vi "FTP Directory check Create if needed.vi"(0 "Host":string, 1 "Create dir":bool, 5 "UserName":string, 7 "Password":string, 9 "PathToCreate":string, 11 "error in (no error)":errorcluster, 12 "timeout ms (60000)":i32=60000) -> (10 "Path":string, 15 "error out":errorcluster)   [LabVIEW 2010]
doc: "This VI checks to see if an FTP file path exists, and if it doesn't then creates it"
uses:
  <vilib>/addons/internet/NI_InternetTK_FTP_VIs.lvlib
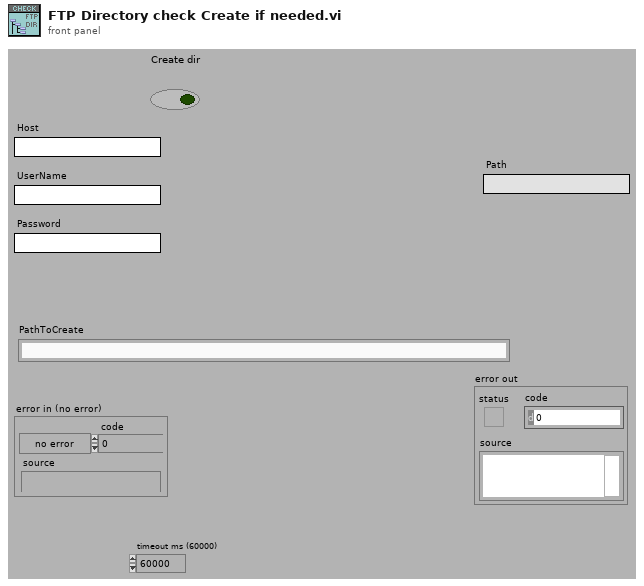
[diagram p1: front panel]
types:
  T1 = typedef "FTP Session.ctl" = refnum<k1>
  T2 = typedef "FTP File Info.ctl" = cluster{"type":enum16{"unknown", "file", "dir", "link"}, "permissions":string, "owner":string, "group":string, "size":i32, "date":string, "name":string, "link name":string}
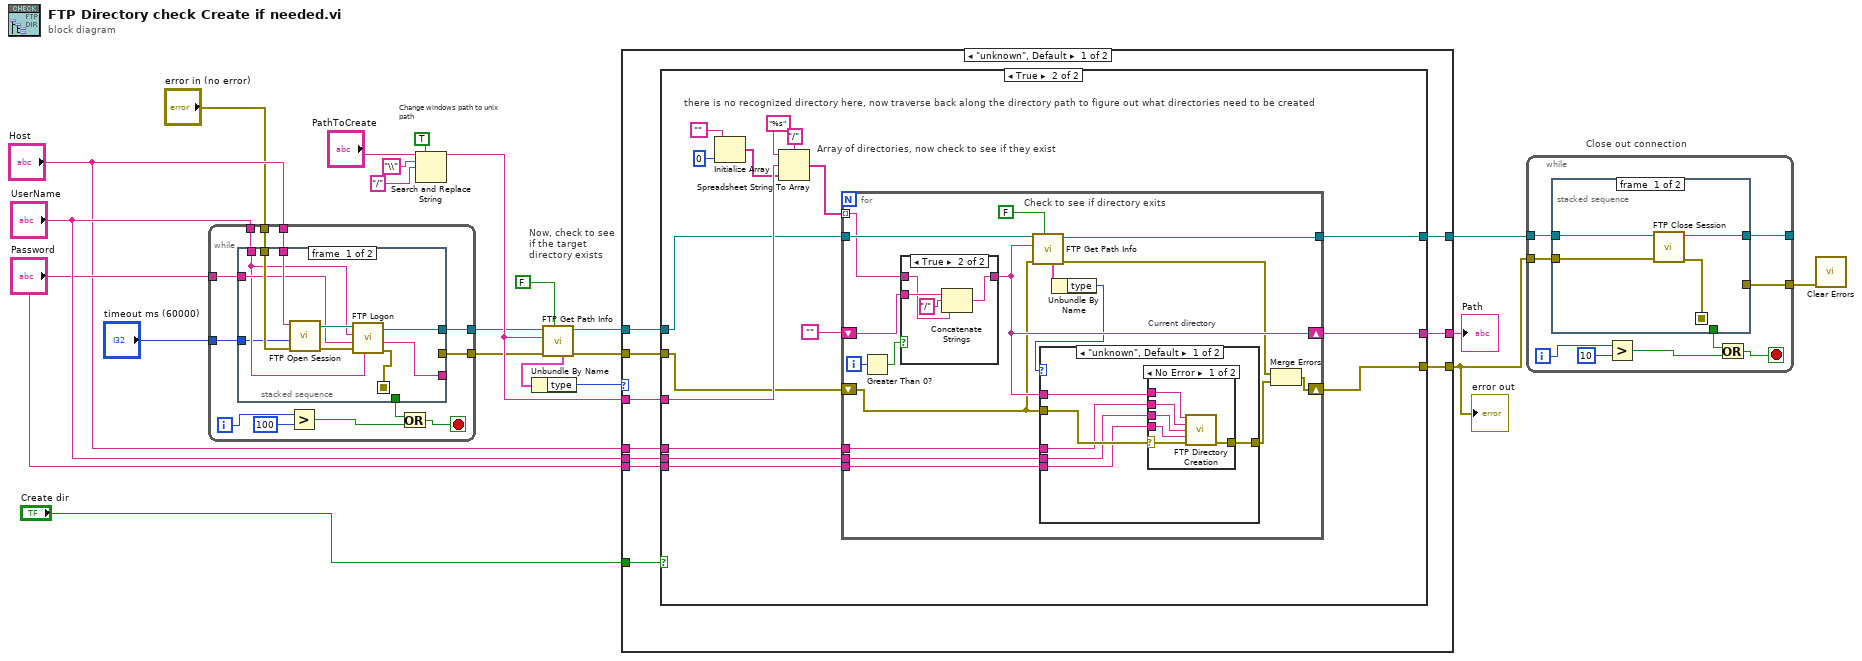
[diagram p0: block diagram]
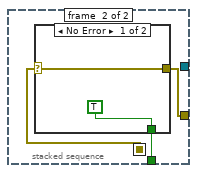
[diagram p2: hidden frame]
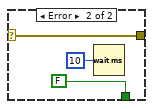
[diagram p3: hidden frame]
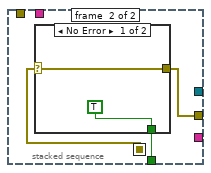
[diagram p4: hidden frame]
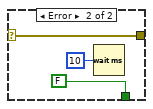
[diagram p5: hidden frame]
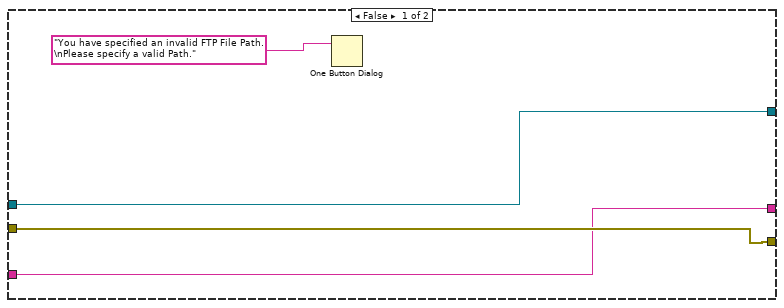
[diagram p6: hidden frame]
diagram:
  # "Close out connection"
  # "Change windows path to unix\npath"
  # "Now, check to see \nif the target \ndirectory exists"
  n1 = while {
    tunnel: [w28] -> w5
    tunnel: [w34] -> w6
    tunnel: "error in (no error)" -> [w33]
    tunnel: "Host" -> [w32]
    tunnel: "Password" -> [w31]
    tunnel: "UserName" -> [w30]
    tunnel: "timeout ms (60000)" -> [w29]
    i -> [w27]
    stop <- w23 stop-if-true
    n2 = stacked-sequence {
      seq-local: [w36 _] -> [_ w47]
      tunnel: [w42 _] -> w34
      tunnel: w33 -> [w41 _]
      tunnel: w32 -> [w40 _]
      tunnel: w31 -> [w39 _]
      tunnel: w30 -> [w38 _]
      tunnel: w29 -> [w37 _]
      tunnel: [_ w46] -> w28
      tunnel: [_ w45] -> w25
      tunnel: [w35 _] -> _
      frame #0 {
        n3 = call <vilib>:"FTP Open Session.vi"("error in (no error)"=w41, "timeout ms (60000)"=w37, "address"=w40) -> ("error out"=w43:errorcluster, "ftp session"=w44:T1)  [unwired: 7 out]
        n4 = call <vilib>:"FTP Logon.vi"("account"=w38, "error in (no error)"=w43, "password"=w39, "user"=w38, "ftp session"=w44) -> ("error out"=w36:errorcluster, "reply string"=w35:string, "ftp session out"=w42:T1)  [unwired: 4 out]
      }
      frame #1 {
        n5 = case shown="No Error" w47 {
          selector: w47 -> [w49 w52]
          tunnel: [w49 w52] -> w46
          tunnel: [TRUE FALSE] -> w45
          frame No Error {
          }
          frame Error {
            n6 = Wait (ms)(milliseconds to wait=u32 10) -> ()  [unwired: 1 out]
          }
        }
      }
    }
    n7 = Greater?(x=w27, y=100) -> (0:w24:bool)
    n8 = Or(x=w25, y=w24) -> (x .or. y?=w23:bool)
  }
  n9 = Search and Replace String(replace all?=TRUE ("replace all? (F)"), input string="PathToCreate", search string="\\", replace string="/" ("replace string (\"\")")) -> (result string=w10:string)  [unwired: 1 in, 6 out]
  n10 = call <vilib>:"FTP Get Path Info.vi"("active (T)"=FALSE, "error in (no error)"=w5, "remote path"=w10, "ftp session"=w6) -> ("error out"=w12:errorcluster, "ftp session out"=w13:T1, "path info"=w8:T2)  [unwired: 5 out]
  n11 = Unbundle By Name(w8) -> ("type"=w9:enum16{"unknown", "file", "dir", "link"})
  n12 = case shown="\"unknown\", Default" w9 {
    tunnel: w10 -> [w62 w121]
    tunnel: [w56 w121] -> w11
    tunnel: w12 -> [w60 w120]
    tunnel: [w54 w120] -> w20
    tunnel: w13 -> [w61 w119]
    tunnel: [w55 w119] -> w21
    tunnel: "Host" -> [w59 _]
    tunnel: "UserName" -> [w58 _]
    tunnel: "Password" -> [w57 _]
    tunnel: "Create dir" -> [w53 _]
    frame "unknown", Default {
      n13 = case shown="True" w53 {
        tunnel: w62 -> [w63 w82]
        tunnel: w61 -> [w65 w75]
        tunnel: w60 -> [w66 w73]
        tunnel: w59 -> [_ w72]
        tunnel: w58 -> [_ w71]
        tunnel: w57 -> [_ w70]
        tunnel: [w63 w69] -> w56
        tunnel: [w65 w68] -> w55
        tunnel: [w66 w67] -> w54
        frame False {
          n14 = One Button Dialog(message="You have specified an invalid FTP File Path.\nPlease specify a valid Path.") -> ()  [unwired: 1 in, 1 out]
        }
        frame True {
          # "Array of directories, now check to see if they exist"
          # "there is no recognized directory here, now traverse back along the directory path to figure out what directories need to be created"
          n15 = Initialize Array("", 0 ("dimension size")) -> (w79:string[])
          n16 = Spreadsheet String To Array(delimiter (Tab)="/", format string="%s", spreadsheet string=w82, array type (2D Dbl)=w79) -> (array=w76:string[])
          n17 = for {
            tunnel: w76 -> [w95] mode=indexing
            shift-right: [w93] -> w69
            shift-left: "" -> [w94]
            tunnel: w75 -> [w98]
            shift-right: [w86] -> w67
            shift-left: w73 -> [w87]
            tunnel: w72 -> [w92]
            tunnel: w71 -> [w91]
            tunnel: w70 -> [w90]
            tunnel: [w89] -> w68
            i -> [w97]
            # "Current directory"
            # "Check to see if directory exits"
            n18 = Greater Than 0?(x=w97) -> (x > 0?=w96:bool)
            n19 = case shown="True" w96 {
              tunnel: w95 -> [w114 w116]
              tunnel: [w114 w115] -> w93
              tunnel: w94 -> [_ w118]
              frame False {
              }
              frame True {
                n20 = Concatenate Strings(w118, "/" ("replace string (\"\")"), w116) -> (w115:string)
              }
            }
            n21 = call <vilib>:"FTP Get Path Info.vi"("active (T)"=FALSE, "error in (no error)"=w87, "remote path"=w93, "ftp session"=w98) -> ("error out"=w84:errorcluster, "ftp session out"=w89:T1, "path info"=w99:T2)  [unwired: 5 out]
            n22 = Unbundle By Name(w99) -> ("type"=w83:enum16{"unknown", "file", "dir", "link"})
            n23 = case shown="\"unknown\", Default" w83 {
              tunnel: w93 -> [w104 _]
              tunnel: w87 -> [w105 w113]
              tunnel: w92 -> [w103 _]
              tunnel: w91 -> [w102 _]
              tunnel: w90 -> [w101 _]
              tunnel: [w100 w113] -> w85
              frame "unknown", Default {
                n24 = case shown="No Error" w105 {
                  selector: w105 -> [w108 w112]
                  tunnel: w104 -> [w110 _]
                  tunnel: w103 -> [w109 _]
                  tunnel: w102 -> [w106 _]
                  tunnel: w101 -> [w107 _]
                  tunnel: [w111 w112] -> w100
                  frame No Error {
                    n25 = call "FTP Directory Creation.vi"("Directory"=w110, "Host"=w109, "User"=w106, "Password"=w107, "error in (no error)"=w108) -> ("error out"=w111:errorcluster)  [unwired: 8 in, 2 out]
                  }
                  frame Error {
                  }
                }
              }
              frame "dir" {
              }
            }
            n26 = Merge Errors(w84, w85) -> (w86:errorcluster)
          }
        }
      }
    }
    frame "dir" {
      # "The directory exists, pass on its path, set ready to true, and quit"
    }
  }
  "Path" <- w11
  "error out" <- w20
  n27 = while {
    tunnel: [w129] -> w22
    tunnel: [w130] -> _
    tunnel: w20 -> [w123]
    tunnel: w21 -> [w122]
    i -> [w128]
    stop <- w124 stop-if-true
    n28 = stacked-sequence {
      seq-local: [w133 _] -> [_ w137]
      tunnel: [w131 _] -> w130
      tunnel: [_ w136] -> w129
      tunnel: [_ w135] -> w126
      tunnel: w123 -> [w134 _]
      tunnel: w122 -> [w132 _]
      frame #0 {
        n29 = call <vilib>:"FTP Close Session.vi"("error in (no error)"=w134, "ftp session"=w132) -> ("error out"=w133:errorcluster, "ftp session out"=w131:T1)  [unwired: 8 out]
      }
      frame #1 {
        n30 = case shown="No Error" w137 {
          selector: w137 -> [w139 w142]
          tunnel: [w139 w142] -> w136
          tunnel: [TRUE FALSE] -> w135
          frame No Error {
          }
          frame Error {
            n31 = Wait (ms)(milliseconds to wait=u32 10) -> ()  [unwired: 1 out]
          }
        }
      }
    }
    n32 = Greater?(x=w128, y=10) -> (0:w125:bool)
    n33 = Or(x=w126, y=w125) -> (x .or. y?=w124:bool)
  }
  n34 = call <vilib>:"Clear Errors.vi"("error in (no error)"=w22) -> ()  [unwired: 6 in, 1 out]
